vi "DPID.Dialog.vi"(8 "error in (no error)":errorcluster, 9 "Existing DPIDs":u8[](array[numeric]), 10 "Existing PIDs":T1[](array[typedef]) {"Signals"."Byte Order" items=["Little Endian", "Big Endian"]; "Signals"."Data Type" items=["Signed", "Unsigned", "IEEE Float"]}, 11 "DPID":T4) -> (0 "error out":errorcluster, 2 "Cancel PID?":bool, 3 "DPID":T4)   [LabVIEW 2019, in "Diagnostics Addon System Explorer.lvlib"]
uses:
  Diagnostics Addon System Explorer.lvlib
  Addon Shared/Types/DPID.Rate.ctl
  Addon Shared/Types/DPID.ctl
  Types/Frame.Export.ctl
  Addon Shared/Types/Signal.ctl
  <vilib>/NI/AMC/Read Termination Message.vi
  <vilib>/NI/AMC/Create Single Message.vi
  <vilib>/NI/AMC/Update Message Routing Info.vi
  <vilib>/NI/AMC/Globals.vi
  <vilib>/NI/AMC/Send Message.vi
  <vilib>/NI/AMC/AMC.lvlib
  Addon Shared/Diagnostics Addon Shared.lvlib
panel:
  in  "Remove":bool
  in  "Speed":T3
  in  "DPID ID":u8=1 min=1 format="%.0x"
  in  "Add":bool
  in  "PID":string(combo)
  in  "PIDs":i32(listbox)
  in  "Cancel PID":bool
  in  "Apply":bool
  in  "Cancel":bool
  in  "OK":bool
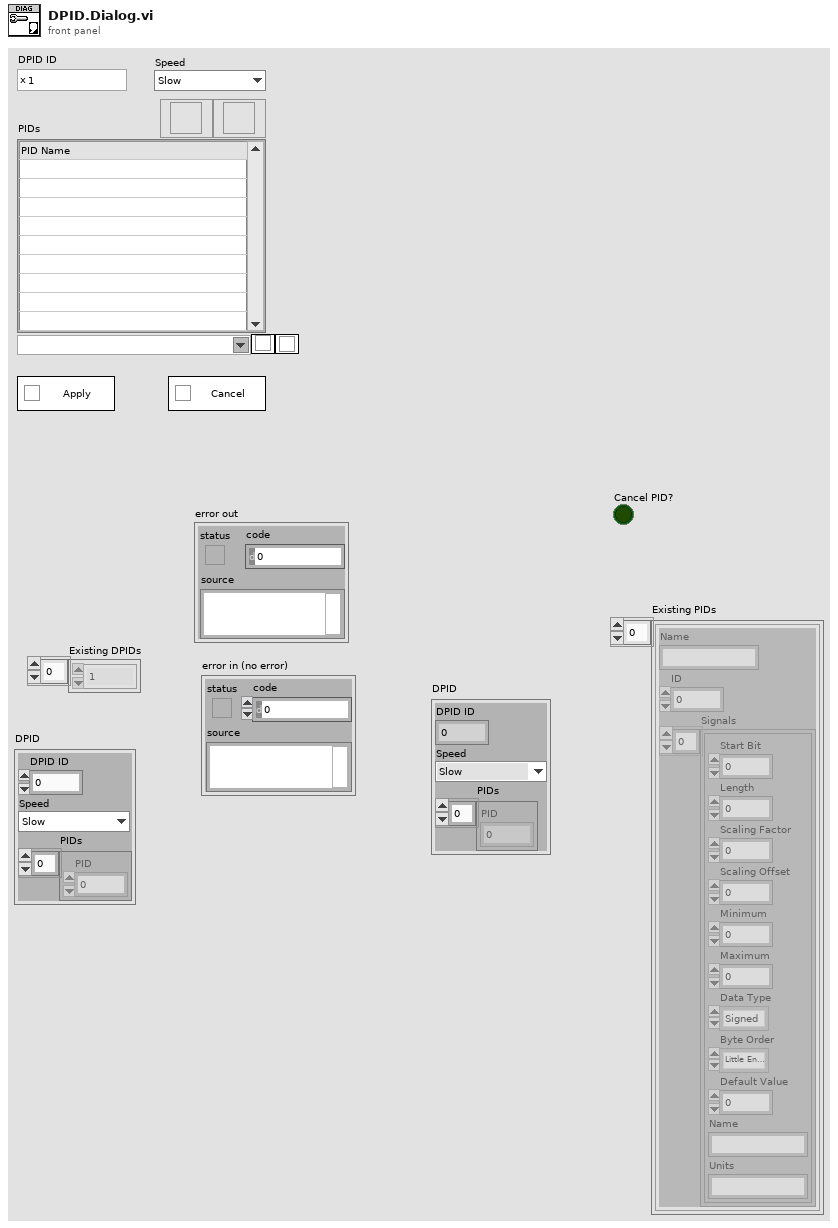
[diagram p1: front panel]
types:
  T1 = typedef "Diagnostics Addon System Explorer.lvlib/Frame.Export.ctl" = cluster{"Name":string, "ID":u32, "Signals":T2[]}
  T2 = typedef "Diagnostics Addon Shared.lvlib/Signal.ctl" = cluster{"Start Bit":u32, "Length":u32, "Scaling Factor":dbl, "Scaling Offset":dbl, "Minimum":dbl, "Maximum":dbl, "Data Type":u32, "Byte Order":u32, "Default Value":dbl, "Name":string, "Units":string}
  T3 = typedef "Diagnostics Addon Shared.lvlib/DPID.Rate.ctl" = enum16{"Slow", "Medium", "Fast"}
  T4 = typedef "Diagnostics Addon Shared.lvlib/DPID.ctl" = cluster{"DPID ID":u8, "Speed":T3, "PIDs":u16[]}
  T5 = cluster{"NewControlRefs":refnum<vi>[], "Add":refnum<vi>, "Listbox":refnum<vi>, "Remove":refnum<vi>, "Apply":refnum<vi>, "Cancel PID":refnum<vi>}
  T6 = typedef "AMC.lvlib/Message Queue.ctl" = refnum<queue>
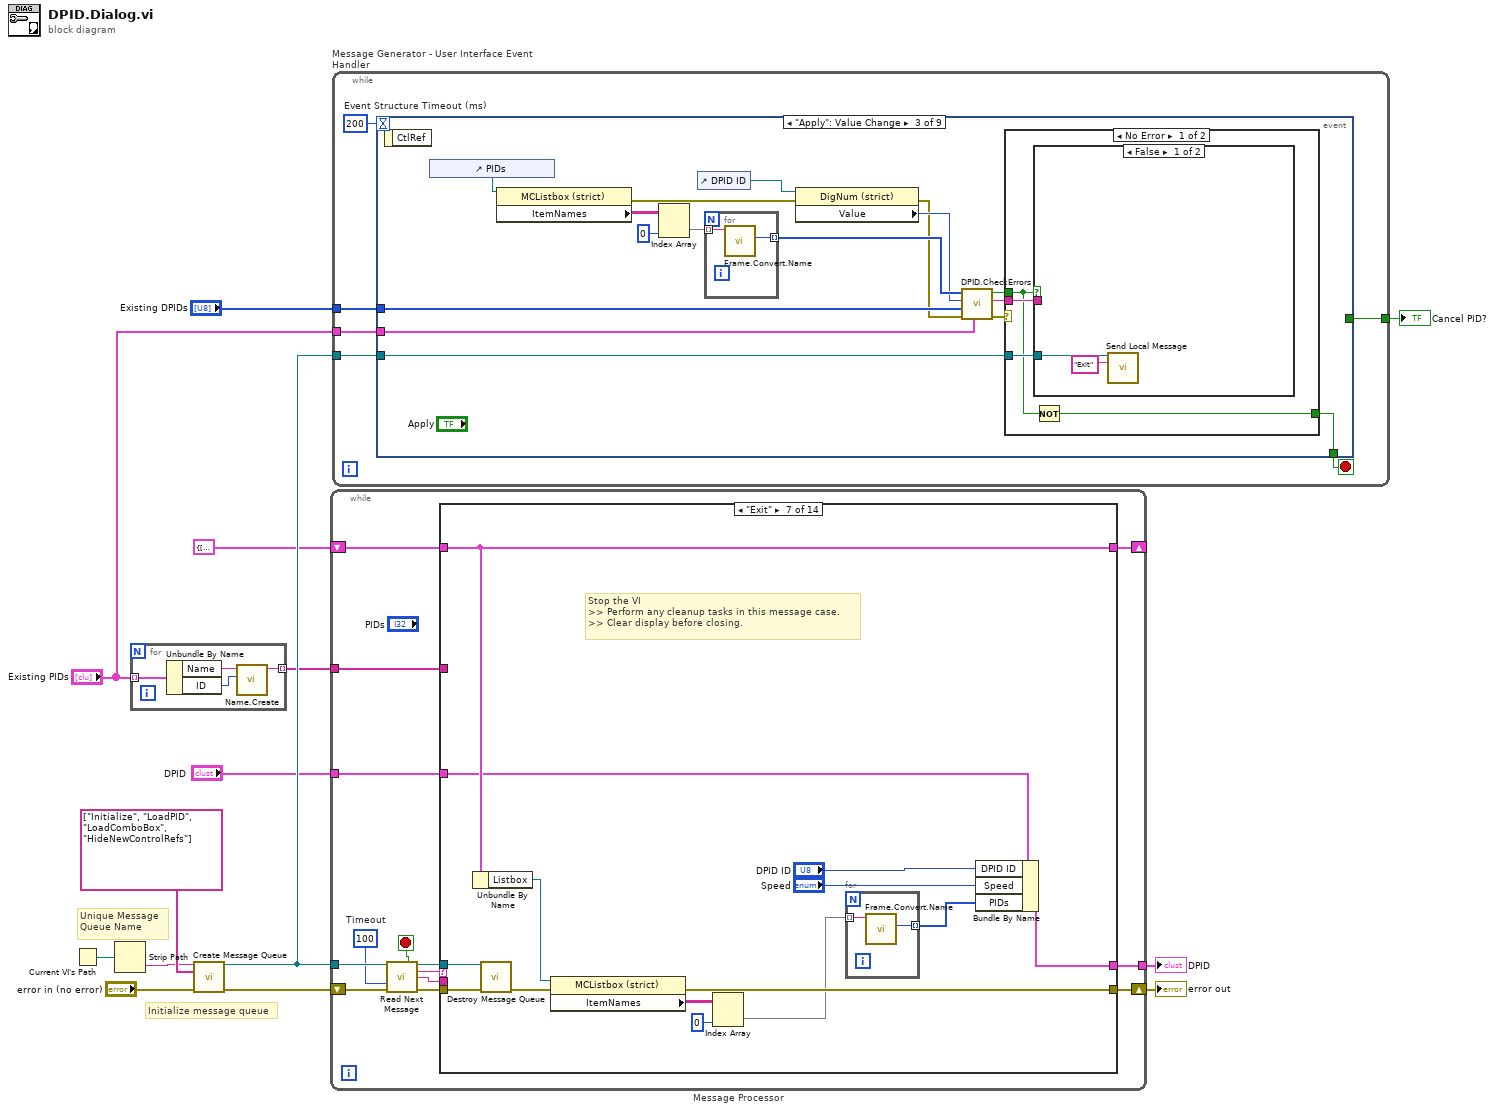
[diagram p0: block diagram]
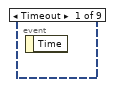
[diagram p2: hidden frame]
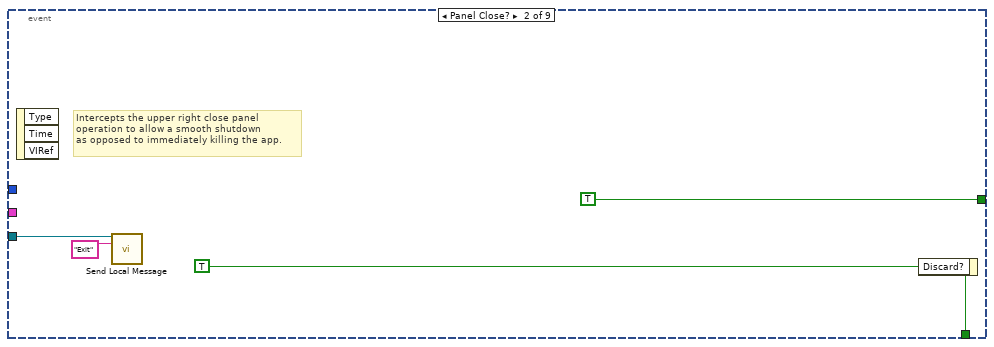
[diagram p3: hidden frame]
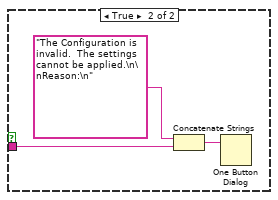
[diagram p4: hidden frame]
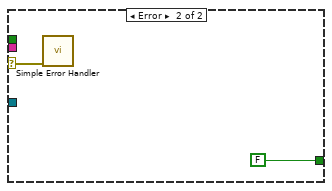
[diagram p5: hidden frame]
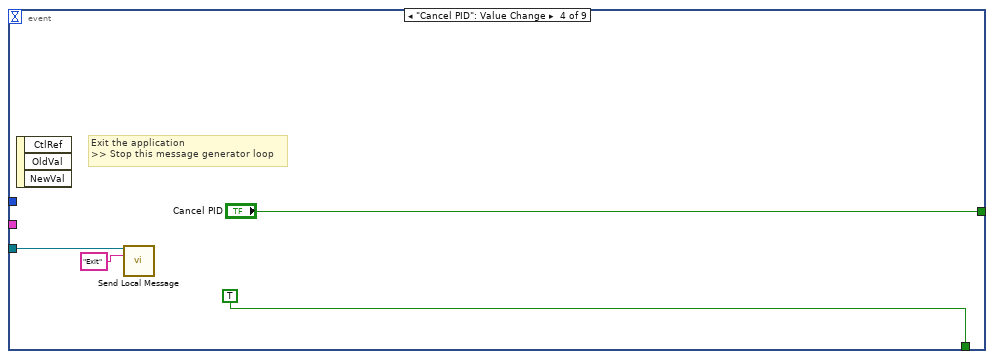
[diagram p6: hidden frame]
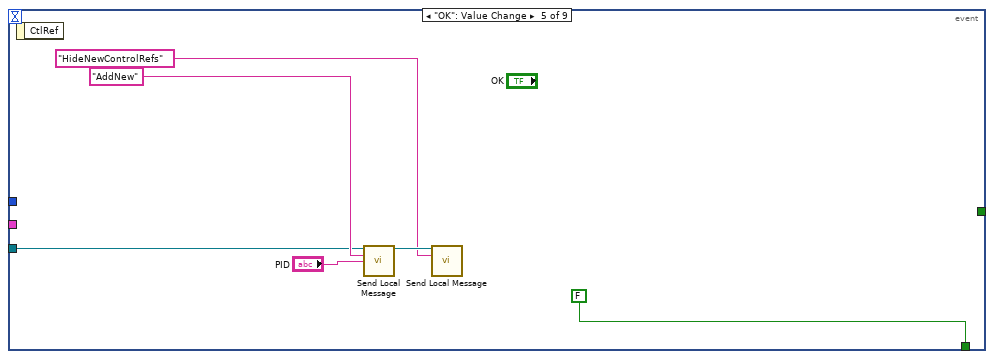
[diagram p7: hidden frame]
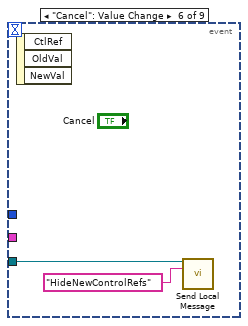
[diagram p8: hidden frame]
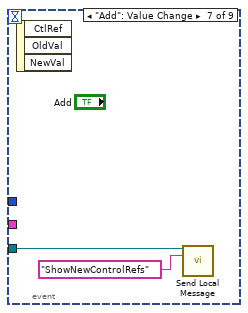
[diagram p9: hidden frame]
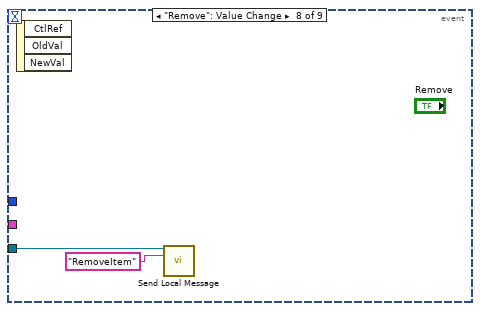
[diagram p10: hidden frame]
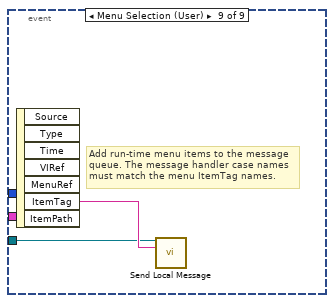
[diagram p11: hidden frame]
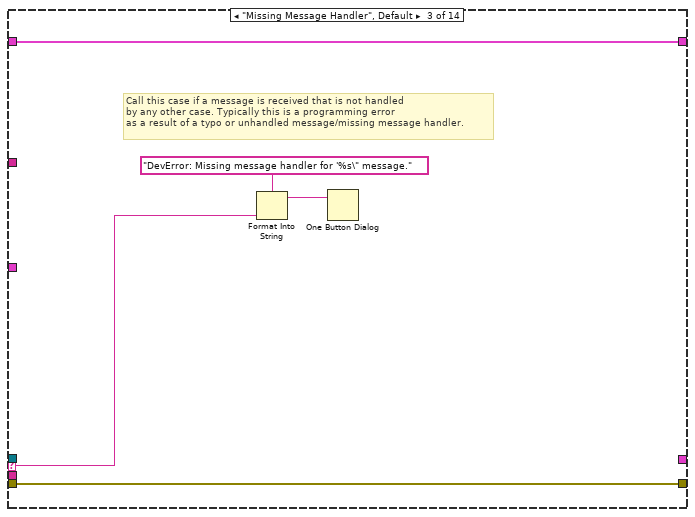
[diagram p14: hidden frame]
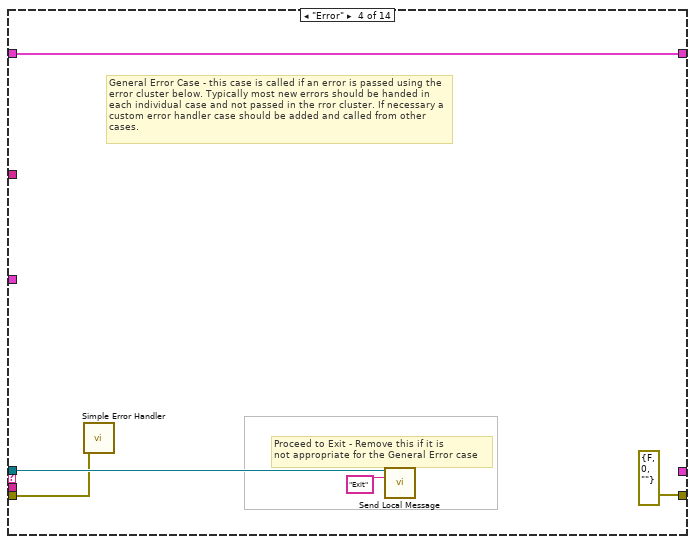
[diagram p15: hidden frame]
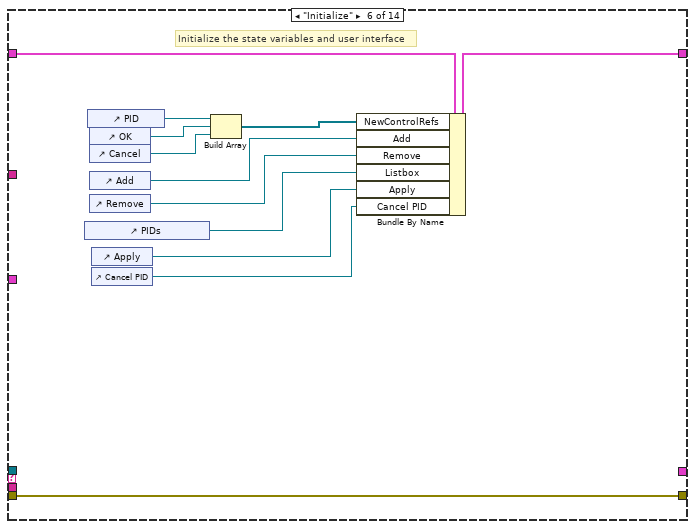
[diagram p17: hidden frame]
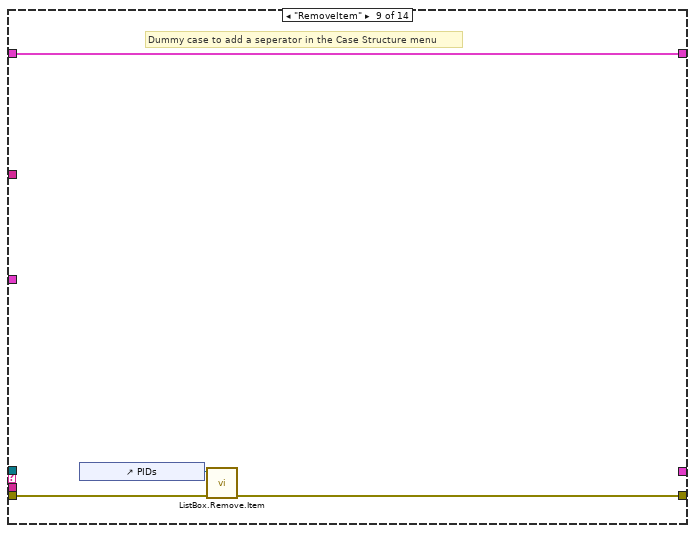
[diagram p19: hidden frame]
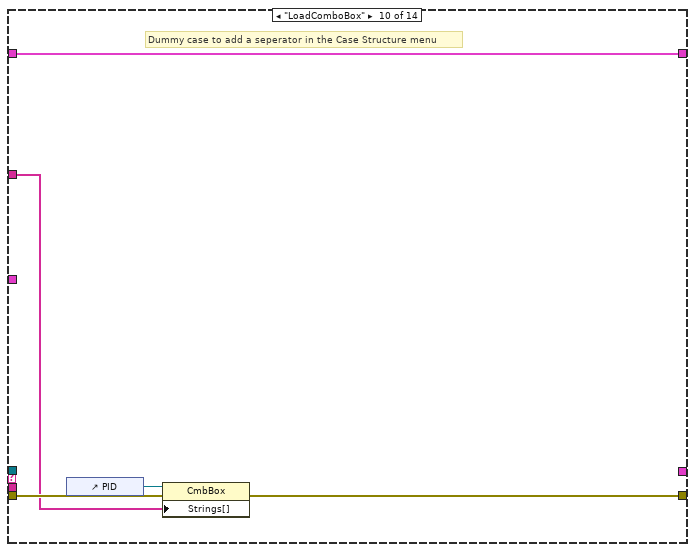
[diagram p20: hidden frame]
diagram:
  # "Initialize message queue"
  # "Unique Message\nQueue Name"
  n1 = Current VI's Path() -> (path=w10:path)
  n2 = Strip Path(path=w10) -> (name=w13:string)  [unwired: 1 out]
  n3 = for {
    tunnel: "Existing PIDs" -> [w18] mode=indexing
    tunnel: [w15] -> w2 mode=indexing
    n4 = Unbundle By Name(w18) -> ("Name"=w16:string, "ID"=w17:u32)
    n5 = call "Name.Create.vi"("PID Number"=w17, "PID Name"=w16) -> ("VS Name"=w15:string)  [unwired: 9 in]
  }
  n6 = call <vilib>:"Create Message Queue.vi"("message queue name"=w13, "initial message names"=string[] ["Initialize", "LoadPID", "LoadComboBox", "HideNewControlRefs"], "error in"="error in (no error)") -> ("message queue out"=w12:T6, "error out"=w11:errorcluster)  [unwired: 11 in]
  n7 = while "Message Processor" {
    shift-left: w11 -> [w26]
    shift-right: [w30] -> w5
    tunnel: w12 -> [w27]
    shift-left: T5 {"NewControlRefs"=[], "Add"=refnum, "Listbox"=refnum, "Remove"=refnum, "Apply"=refnum, "Cancel PID"=refnum} ("State Variables") -> [w32]
    shift-right: [w31] -> _
    tunnel: [w21] -> w7
    tunnel: "DPID" -> [w20]
    tunnel: w2 -> [w19]
    stop <- w29 stop-if-true
    w24 = 100  # Timeout
    n8 = call <vilib>:"Read Next Message.vi"("message queue in"=w27, "timeout (1 ms)"=w24, "error in"=w26) -> ("exit process?"=w29:bool, "message queue out"=w28:T6, "message name"=w23:string, "message value"=w22:string, "error out"=w25:errorcluster)  [unwired: 5 in, 3 out]
    n9 = case shown="\"Exit\"" w23 {
      selector: w23 -> [_ _ w39 _ _ _ _ _ _ _ _ _ _ _]
      tunnel: [w34 w36 w41 w46 w48 w55 w72 w78 w82 w87 w105 w125 w139 w154] -> w31
      tunnel: w32 -> [w34 w36 w41 w46 w48 w56 w72 w78 w82 w87 w105 w125 w139 w154]
      tunnel: w28 -> [_ _ _ w44 _ _ w73 _ _ _ _ _ _ _]
      tunnel: w25 -> [w33 w35 w40 w42 w47 w53 w74 w77 w80 w85 w99 w122 w138 w153]
      tunnel: [w33 w35 w40 errorcluster {"status"=FALSE, "code"=0, "source"=""} ("error out") w47 w53 w65 w77 w79 w84 w98 w123 w129 w142] -> w30
      tunnel: w22 -> [_ _ _ _ _ _ _ _ _ _ _ w121 _ _]
      tunnel: [_ _ _ _ _ _ w68 _ _ _ _ _ _ _] -> w21
      tunnel: w20 -> [_ _ _ _ _ _ w67 _ _ _ w97 _ _ _]
      tunnel: w19 -> [_ _ _ _ _ _ _ _ _ w83 w88 _ _ _]
      frame "---------- Framework Operations ----------" {
        # "Dummy case to add a seperator in the Case Structure menu"
      }
      frame "", "Idle" {
        # "Idle Case - this case is called after a Timeout on the Get Next Message from Queue VI, if no new messages are present on the queue. This case can be used for housekeeping tasks such as updating the UI."
      }
      frame "Missing Message Handler", Default {
        # "Call this case if a message is received that is not handled \nby any other case. Typically this is a programming error\nas a result of a typo or unhandled message/missing message handler."
        n10 = Format Into String(format string="DevError: Missing message handler for '%s\" message." ("message"), w39) -> (resulting string=w37:string)  [unwired: 2 in, 1 out]
        n11 = One Button Dialog(message=w37) -> ()  [unwired: 2 out]
      }
      frame "Error" {
        # "Proceed to Exit - Remove this if it is\nnot appropriate for the General Error case"
        # "General Error Case - this case is called if an error is passed using the error cluster below. Typically most new errors should be handed in each individual case and not passed in the rror cluster. If necessary a custom error handler case should be added and called from other cases."
        n12 = call <vilib>:"Simple Error Handler.vi"("error in (no error)"=w42) -> ()  [unwired: 1 in, 8 out]
        n13 = call <vilib>:"Send Local Message.vi"("message queue in"=w44, "message name"="Exit") -> ()  [unwired: 11 in, 3 out]
      }
      frame "---------- Generic Operations ----------" {
        # "Dummy case to add a seperator in the Case Structure menu"
      }
      frame "Initialize" {
        # "Initialize the state variables and user interface"
        n14 = control-ref of="PIDs"() -> (w54:refnum<vi>)
        n15 = control-ref of="PID"() -> (w58:refnum<vi>)
        n16 = control-ref of="OK"() -> (w59:refnum<vi>)
        n17 = control-ref of="Cancel"() -> (w60:refnum<vi>)
        n18 = control-ref of="Add"() -> (w52:refnum<vi>)
        n19 = control-ref of="Remove"() -> (w51:refnum<vi>)
        n20 = control-ref of="Apply"() -> (w50:refnum<vi>)
        n21 = control-ref of="Cancel PID"() -> (w49:refnum<vi>)
        n22 = Build Array(w58, w59, w60) -> (w57:refnum<vi>[])
        n23 = Bundle By Name(cluster=w56, "NewControlRefs"=w57, "Add"=w52, "Remove"=w51, "Listbox"=w54, "Apply"=w50, "Cancel PID"=w49) -> (w55:T5)
      }
      frame "Exit" {
        # "Stop the VI\n>> Perform any cleanup tasks in this message case.\n>> Clear display before closing."
        n24 = Unbundle By Name(w72) -> ("Listbox"=w71:refnum<vi>)
        n25 = call <vilib>:"Destroy Message Queue.vi"("message queue in"=w73, "error in"=w74) -> ("error out"=w70:errorcluster)  [unwired: 11 in, 2 out]
        n26 = property class="MCListbox (strict)"(reference=w71, error in=w70) -> (error out=w65:errorcluster, "ItemNames"=w66:string[][])  [unwired: 1 out]
        n27 = Index Array(array=w66, index (col)=0 ("disabled index (col)")) -> (element=w61:string[])  [unwired: 1 in]
        n28 = for {
          tunnel: w61 -> [w75] mode=indexing
          tunnel: [w76] -> w62 mode=indexing
          n29 = call "Frame.Convert.Name.vi"("VS Frame Name"=w75) -> ("ID"=w76:u16)  [unwired: 9 in, 1 out]
        }
        n30 = Bundle By Name(cluster=w67, "DPID ID"="DPID ID", "Speed"="Speed", "PIDs"=w62) -> (w68:T4)
      }
      frame "---------- Application Operations ----------" {
        # "Dummy case to add a seperator in the Case Structure menu"
      }
      frame "RemoveItem" {
        # "Dummy case to add a seperator in the Case Structure menu"
        n31 = control-ref of="PIDs"() -> (w81:refnum<vi>)
        n32 = call "ListBox.Remove.Item.vi"("error in (no error)"=w80, "MulticolumnListbox in"=w81) -> ("error out"=w79:errorcluster)  [unwired: 9 in]
      }
      frame "LoadComboBox" {
        # "Dummy case to add a seperator in the Case Structure menu"
        n33 = control-ref of="PID"() -> (w86:refnum<vi>)
        n34 = property class="CmbBox"(reference=w86, error in=w85, "Strings[]"=w83) -> (error out=w84:errorcluster)  [unwired: 1 out]
      }
      frame "LoadPID" {
        # "Dummy case to add a seperator in the Case Structure menu"
        n35 = Unbundle By Name(w97) -> ("PIDs"=w91:u16[], "Speed"=w95:T3, "DPID ID"=w96:u8)
        n36 = for {
          tunnel: w88 -> [w118] mode=indexing
          tunnel: [w119] -> w92 mode=indexing
          n37 = call "Frame.Convert.Name.vi"("VS Frame Name"=w118) -> ("ID"=w119:u16)  [unwired: 9 in, 1 out]
        }
        n38 = control-ref of="DPID ID"() -> (w101:refnum<vi>)
        n39 = control-ref of="Speed"() -> (w94:refnum<vi>)
        n40 = for {
          tunnel: w92 -> [w110]
          tunnel: w88 -> [w109]
          tunnel: w91 -> [w106] mode=indexing
          tunnel: [w108] -> w90 mode=indexing
          n41 = Search 1D Array(1D array=w110, element=w106) -> (index of element=w107:i32)  [unwired: 1 in]
          n42 = case shown="Default" w107 {
            selector: w107 -> [_ w115]
            tunnel: w109 -> [_ w117]
            tunnel: [w111 w116] -> w108
            tunnel: w106 -> [w114 _]
            frame -1 {
              n43 = Number To Hexadecimal String(2:w114) -> (0:w113:string)  [unwired: 1 in]
              n44 = Concatenate Strings(w113, " - Error: No Matching PID" ("PID Name")) -> (w111:string)
            }
            frame Default {
              n45 = Index Array(array=w117, index=w115) -> (element=w116:string)
            }
          }
        }
        n46 = property class="DigNum (strict)"(reference=w101, error in=w99, "Value"=w96) -> (error out=w102:errorcluster)  [unwired: 1 out]
        n47 = property class="Enum (strict)"(reference=w94, error in=w102, "Value"=w95) -> (error out=w100:errorcluster)  [unwired: 1 out]
        n48 = control-ref of="PIDs"() -> (w104:refnum<vi>)
        n49 = Build Array(w90) -> (w89:string[][])
        n50 = Transpose 2D Array(2D array=w89) -> (transposed array=w93:string[][])
        n51 = property class="MCListbox (strict)"(reference=w104, error in=w100, "ItemNames"=w93, "Value"=0) -> (error out=w98:errorcluster)  [unwired: 1 out]
      }
      frame "AddNew" {
        # "Dummy case to add a seperator in the Case Structure menu"
        n52 = Build Array(w121) -> (w120:string[])
        n53 = Unbundle By Name(w125) -> ("Listbox"=w124:refnum<vi>)
        n54 = call "Listbox.Add.Item.vi"("error in (no error)"=w122, "Item"=w120, "MulticolumnListbox in"=w124) -> ("error out"=w123:errorcluster)  [unwired: 8 in]
      }
      frame "HideNewControlRefs" {
        w126 = TRUE ("Visible")
        # "Dummy case to add a seperator in the Case Structure menu"
        n55 = Unbundle By Name(w139) -> ("Cancel PID"=w127:refnum<vi>, "Apply"=w128:refnum<vi>, "Remove"=w132:refnum<vi>, "Add"=w134:refnum<vi>, "NewControlRefs"=w137:refnum<vi>[])
        n56 = call "Controls.Set.Visible.vi"("error in"=w138, "Visible?"=FALSE, "Control Refs"=w137) -> ("error out"=w135:errorcluster)  [unwired: 8 in]
        n57 = property class="Bool"(reference=w134, error in=w135, "Visible"=w126) -> (error out=w133:errorcluster)  [unwired: 1 out]
        n58 = property class="Bool"(reference=w132, error in=w133, "Visible"=w126) -> (error out=w130:errorcluster)  [unwired: 1 out]
        n59 = property class="Bool"(reference=w128, error in=w130, "Visible"=w126) -> (error out=w131:errorcluster)  [unwired: 1 out]
        n60 = property class="Bool"(reference=w127, error in=w131, "Visible"=w126) -> (error out=w129:errorcluster)  [unwired: 1 out]
      }
      frame "ShowNewControlRefs" {
        w145 = FALSE ("Visible")
        w147 = FALSE ("Visible")
        # "Dummy case to add a seperator in the Case Structure menu"
        n61 = Unbundle By Name(w154) -> ("Apply"=w141:refnum<vi>, "Cancel PID"=w140:refnum<vi>, "Remove"=w146:refnum<vi>, "Add"=w149:refnum<vi>, "NewControlRefs"=w152:refnum<vi>[])
        n62 = call "Controls.Set.Visible.vi"("error in"=w153, "Visible?"=TRUE, "Control Refs"=w152) -> ("error out"=w150:errorcluster)  [unwired: 8 in]
        n63 = property class="Bool"(reference=w149, error in=w150, "Visible"=w147) -> (error out=w148:errorcluster)  [unwired: 1 out]
        n64 = property class="Bool"(reference=w146, error in=w148, "Visible"=w147) -> (error out=w143:errorcluster)  [unwired: 1 out]
        n65 = property class="Bool"(reference=w140, error in=w143, "Visible"=w145) -> (error out=w144:errorcluster)  [unwired: 1 out]
        n66 = property class="Bool"(reference=w141, error in=w144, "Visible"=w145) -> (error out=w142:errorcluster)  [unwired: 1 out]
      }
    }
  }
  "DPID" <- w7
  "error out" <- w5
  n67 = while "Message Generator - User Interface Event Handler" {
    tunnel: w12 -> [w158]
    tunnel: [w157] -> w8
    tunnel: "Existing DPIDs" -> [w156]
    tunnel: "Existing PIDs" -> [w155]
    stop <- w159 stop-if-true
    w160 = 200  # Event Structure Timeout (ms)
    n68 = event shown="[2] \"Apply\": Value Change" {
      selector: _ -> [_ _ _ _ _ _ _ _ _]
      dyn-events: _ -> [_ _ _ _ _ _ _ _ _]
      timeout: w160 -> [_ _ _ _ _ _ _ _ _]
      tunnel: [_ w164 w174 TRUE ("Discard?") FALSE ("Discard?") _ _ _ _] -> w159
      tunnel: w158 -> [_ w162 w178 w195 w201 w204 w206 w208 w210]
      tunnel: [_ TRUE ("Cancel PID") _ "Cancel PID" _ _ _ _ _] -> w157
      tunnel: w156 -> [_ _ w180 _ _ _ _ _ _]
      tunnel: w155 -> [_ _ w179 _ _ _ _ _ _]
      event Timeout {
        n69 = event-data() -> ()  [unwired: 2 out]
      }
      event Panel Close? {
        w164 = TRUE ("Discard?")
        # "Intercepts the upper right close panel\noperation to allow a smooth shutdown\nas opposed to immediately killing the app."
        n70 = event-data() -> ()  [unwired: 4 out]
        n71 = call <vilib>:"Send Local Message.vi"("message queue in"=w162, "message name"="Exit") -> ()  [unwired: 11 in, 3 out]
        n72 = event-data("Discard?"=w164) -> ()  [unwired: 1 in, 1 out]
      }
      event "Apply": Value Change {
        n73 = event-data() -> ()  [unwired: 2 out]
        n74 = control-ref of="PIDs"() -> (w170:refnum<vi>)
        n75 = property class="MCListbox (strict)"(reference=w170) -> (error out=w166:errorcluster, "ItemNames"=w173:string[][])  [unwired: 1 in, 1 out]
        n76 = Index Array(array=w173, index (col)=0 ("disabled index (col)")) -> (element=w171:string[])  [unwired: 1 in]
        n77 = control-ref of="DPID ID"() -> (w168:refnum<vi>)
        n78 = for {
          tunnel: w171 -> [w181] mode=indexing
          tunnel: [w182] -> w169 mode=indexing
          n79 = call "Frame.Convert.Name.vi"("VS Frame Name"=w181) -> ("ID"=w182:u16)  [unwired: 9 in, 1 out]
        }
        n80 = property class="DigNum (strict)"(reference=w168, error in=w166) -> (error out=w165:errorcluster, "Value"=w167:u8)  [unwired: 1 out]
        n81 = call "DPID.CheckErrors.vi"("Existing PIDs"=w179, "error in (no error)"=w165, "Existing DPIDs"=w180, "DPID ID"=w167, "PIDs"=w169) -> ("error out"=w176:errorcluster, "Reason"=w175:string, "Error?"=w177:bool)  [unwired: 4 in]
        n82 = case shown="No Error" w176 {
          selector: w176 -> [_ w193]
          tunnel: w177 -> [w184 _]
          tunnel: w178 -> [w186 _]
          tunnel: w175 -> [w185 _]
          tunnel: [w183 FALSE] -> w174
          frame No Error {
            n83 = case shown="False" w184 {
              tunnel: w186 -> [w188 _]
              tunnel: w185 -> [_ w191]
              frame False {
                n84 = call <vilib>:"Send Local Message.vi"("message queue in"=w188, "message name"="Exit" ("Message Name")) -> ()  [unwired: 11 in, 3 out]
              }
              frame True {
                n85 = Concatenate Strings("The Configuration is invalid.  The settings cannot be applied.\n\nReason:\n" ("message"), w191) -> (w189:string)
                n86 = One Button Dialog(message=w189) -> ()  [unwired: 1 in, 1 out]
              }
            }
            n87 = Not(x=w184) -> (.not. x?=w183:bool)
          }
          frame Error {
            n88 = call <vilib>:"Simple Error Handler.vi"("error in (no error)"=w193) -> ()  [unwired: 4 in, 5 out]
          }
        }
      }
      event "Cancel PID": Value Change {
        # "Exit the application\n>> Stop this message generator loop"
        n89 = event-data() -> ()  [unwired: 4 out]
        n90 = call <vilib>:"Send Local Message.vi"("message queue in"=w195, "message name"="Exit") -> ()  [unwired: 11 in, 3 out]
      }
      event "OK": Value Change {
        n91 = event-data() -> ()  [unwired: 2 out]
        n92 = call <vilib>:"Send Local Message.vi"("message queue in"=w201, "message name"="AddNew", "message value"="PID") -> ("message queue out"=w200:T6)  [unwired: 10 in, 2 out]
        n93 = call <vilib>:"Send Local Message.vi"("message queue in"=w200, "message name"="HideNewControlRefs" ("Message Name")) -> ()  [unwired: 11 in, 3 out]
      }
      event "Cancel": Value Change {
        n94 = event-data() -> ()  [unwired: 4 out]
        n95 = call <vilib>:"Send Local Message.vi"("message queue in"=w204, "message name"="HideNewControlRefs" ("Message Name")) -> ()  [unwired: 11 in, 3 out]
      }
      event "Add": Value Change {
        n96 = event-data() -> ()  [unwired: 4 out]
        n97 = call <vilib>:"Send Local Message.vi"("message queue in"=w206, "message name"="ShowNewControlRefs" ("Message Name")) -> ()  [unwired: 11 in, 3 out]
      }
      event "Remove": Value Change {
        n98 = event-data() -> ()  [unwired: 4 out]
        n99 = call <vilib>:"Send Local Message.vi"("message queue in"=w208, "message name"="RemoveItem") -> ()  [unwired: 11 in, 3 out]
      }
      event Menu Selection (User) {
        # "Add run-time menu items to the message\nqueue. The message handler case names must match the menu ItemTag names."
        n100 = event-data() -> ("ItemTag"=w211:string)  [unwired: 7 out]
        n101 = call <vilib>:"Send Local Message.vi"("message queue in"=w210, "message name"=w211) -> ()  [unwired: 11 in, 3 out]
      }
    }
  }
  "Cancel PID?" <- w8
